vi "GetLowPrioritySensors.vi"() -> ()   [LabVIEW 2023]
doc: "All low priority sensor reads should be placed in this VI."
uses:
  GlobalNoteHandling.vi
  GlobalMiscellaneous.vi
  GlobalDriverStationData.vi
  GlobalDrivebase.vi
  GRNF_CTREMotor.vi
  <vilib>/Rock Robotics/WPI/ThirdParty/Phoenix-LabVIEW/Motor Controller/Get/CTRE_Phoenix_MotorController_GetTemperature.vi
  GRNF_Compressor.vi
  GlobalElevator.vi
  GlobalShooter.vi
  GRNF_GenericMotor.vi
  GRNF_Kraken.vi
  <vilib>/Rock Robotics/WPI/ThirdParty/Phoenix6/getters/GetPRO_SupplyAndTemp_DeviceTemp.vi
  <vilib>/Rock Robotics/WPI/ThirdParty/Phoenix6/getters/GetPRO_RotorPosAndVel_Velocity.vi
panel:
  out "Pressure Change (psi/min)":dbl
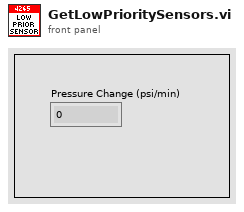
[diagram p1: front panel]
types:
  T1 = typedef "DeviceReference.ctl" = cluster{"CANbus Name":string, "Device Encoding":u32, "Device Name":string}
  T2 = cluster{"Value":dbl, "System Timestamp":dbl, "CANivore Timestamp":dbl, "ECU Timestamp":dbl}
  T3 = typedef "WPI_MotorControlDeviceRef.ctl" = cluster{"DeviceStatus":errorcluster, "Type":T4, "PWM":cluster{"PWM Channel":T5, "DeadBand":T6}, "CAN":cluster{"Device Number":u8, "SetOutput VI Ref":variant, "GetOutput VI Ref":variant, "Enable VI Ref":variant, "Disable VI Ref":variant, "Data":variant}, "Invert":bool, "DIO PWM":cluster{"PWM \"Enable\" Channel":T5, "DIOChannel":T7, "PWM Rate":dbl}}
  T4 = typedef "WPI_MotorControlType.ctl" = enum16{"PWM", "CAN", "DIO PWM"}
  T5 = typedef "FPGA_DIOPWMChannel.ctl" = enum8{"PWM 0", "PWM 1", "PWM 2", "PWM 3", "PWM 4", "PWM 5", "PWM 6", "PWM 7", "PWM 8", "PWM 9", "PWM MXP 0", "PWM MXP 1", "PWM MXP 2", "PWM MXP 3", "PWM MXP 4", "PWM MXP 5", "PWM MXP 6", "PWM MXP 7", "PWM MXP 8", "PWM MXP 9", "Invalid"}
  T6 = typedef "WPI_PWMDeadband.ctl" = cluster{"Name":string, "maxPositivePwm":i32, "minPositivePwm":i32, "centerPwm":i32, "maxNegativePwm":i32, "minNegativePwm":i32, "angularRange":u16}
  T7 = typedef "FPGA_DIOChannel.ctl" = enum8{"DIO 0", "DIO 1", "DIO 2", "DIO 3", "DIO 4", "DIO 5", "DIO 6", "DIO 7", "DIO 8", "DIO 9", "DIO MXP 0", "DIO MXP 1", "DIO MXP 2", "DIO MXP 3", "DIO MXP 4", "DIO MXP 5", "DIO MXP 6", "DIO MXP 7", "DIO MXP 8", "DIO MXP 9", "DIO MXP 10", "DIO MXP 11", "DIO MXP 12", "DIO MXP 13", "DIO MXP 14", "DIO MXP 15", "SPI Port CS1", "SPI Port CS2", "SPI Port CS3", "SPI Port MISO", "SPI Port MOSI", "Invalid"}
  T8 = typedef "WPI_CompressorDevRef.ctl" = cluster{"DevStatus":errorcluster, "Pneumatics Control Module":u8}
  T9 = cluster{"Pressure 0 (psi)":dbl, "Pressure 1 (psi)":dbl}
  T10 = cluster{"Battery Voltage Fault":bool, "Hardware Fault":bool, "CAN Warning Fault":bool, "Temperature Fault":bool}
  T11 = cluster{"HardwareFault":bool, "CompressorFault":bool, "SolenoidFault":bool, "Compressor Open":bool, "Brownout":bool}
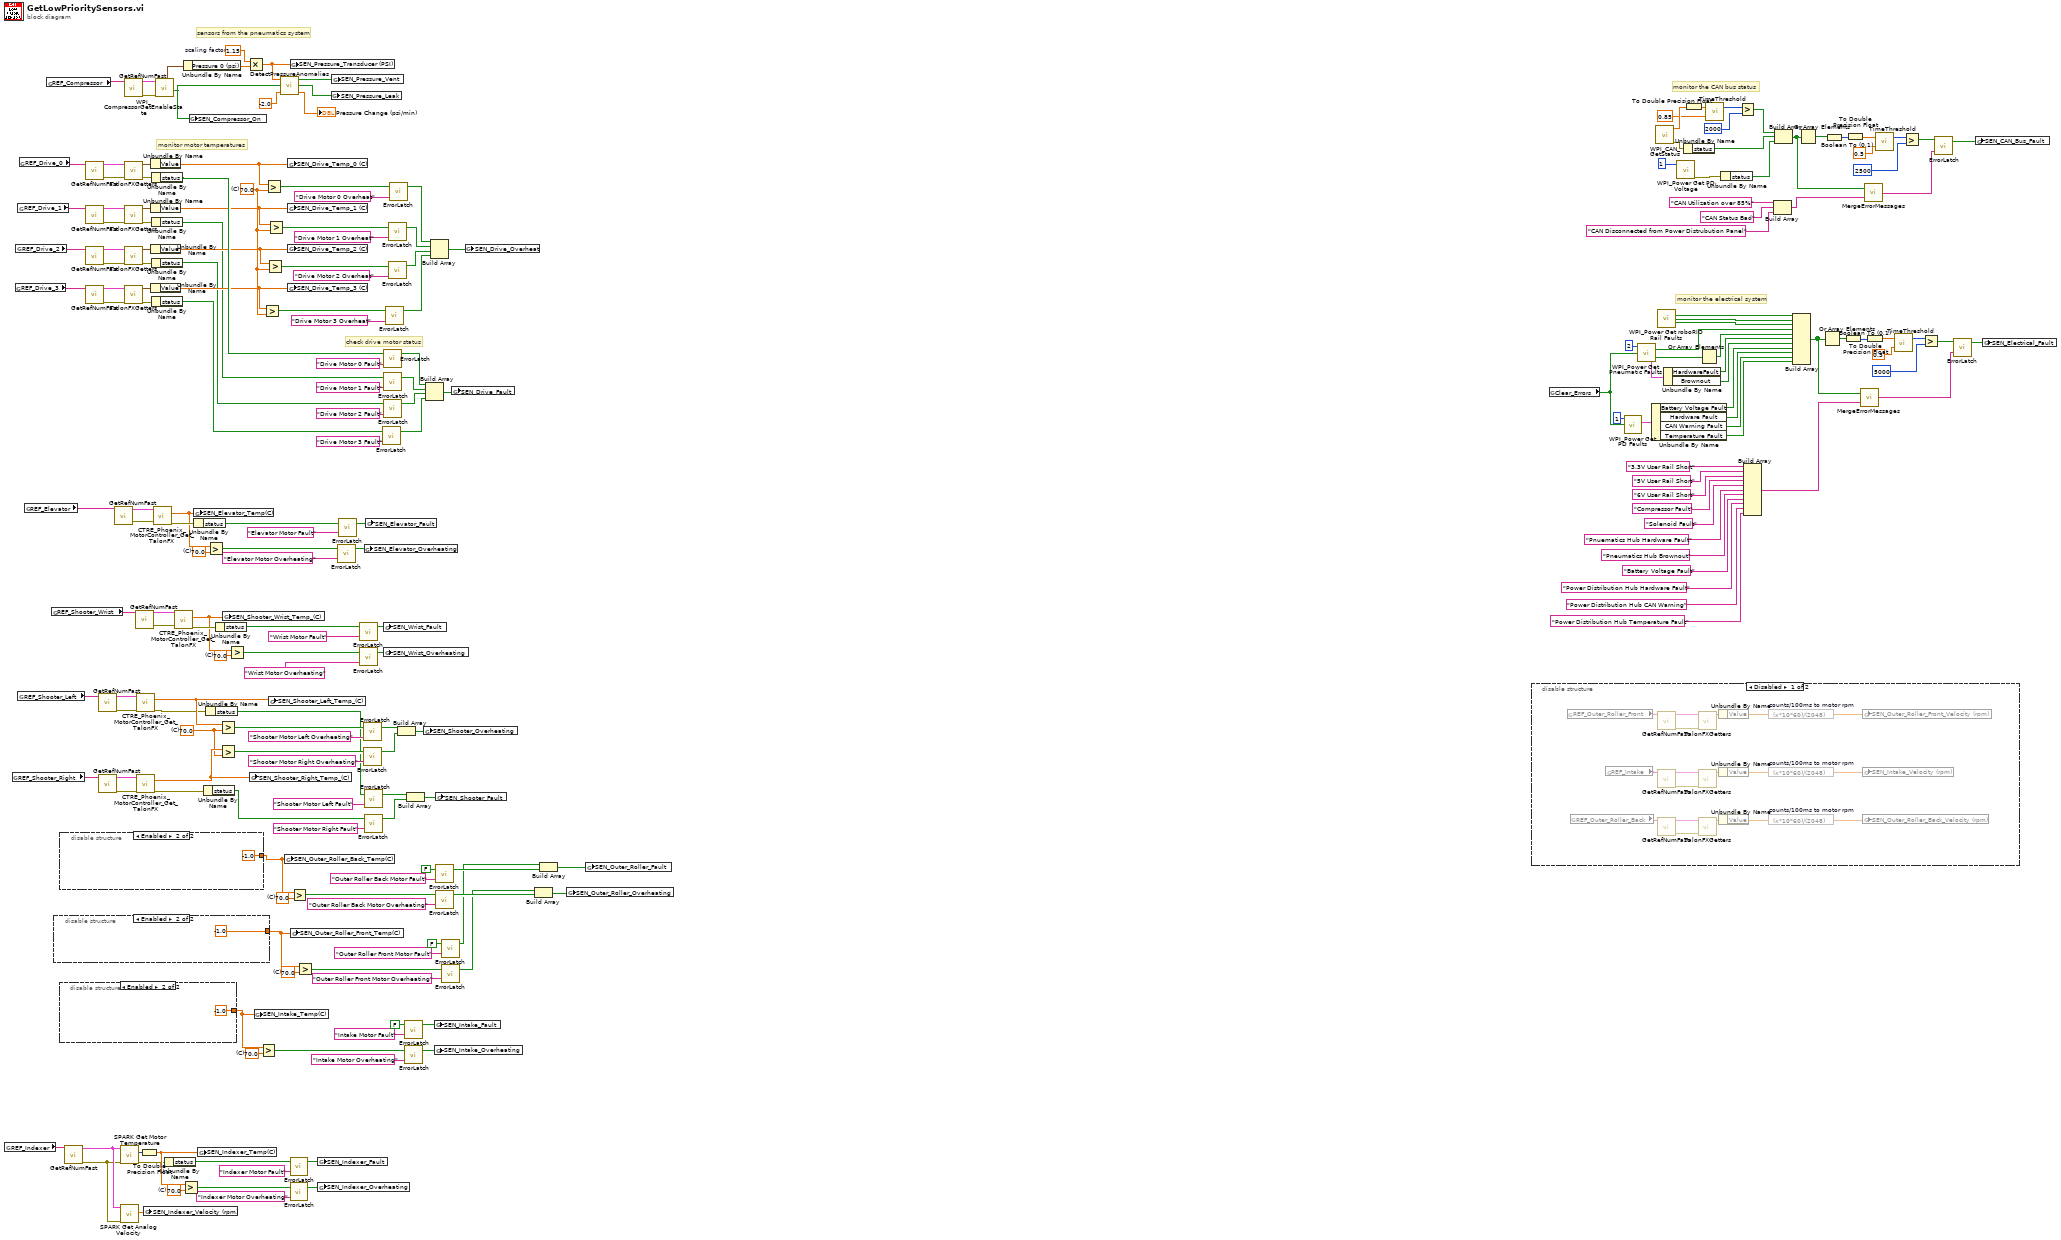
[diagram p0: block diagram]
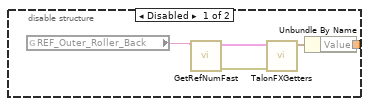
[diagram p3: hidden frame]
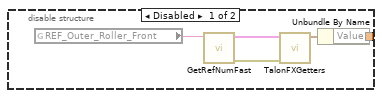
[diagram p4: hidden frame]
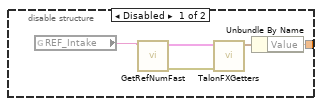
[diagram p5: hidden frame]
diagram:
  w34 = 70.0  # (C)
  w42 = 70.0  # (C)
  w49 = 70.0  # (C)
  w60 = 70.0  # (C)
  w78 = 70.0  # (C)
  w105 = 70.0  # (C)
  w108 = 70.0  # (C)
  w129 = 1.15  # scaling factor
  w216 = 70.0  # (C)
  # "check drive motor status"
  # "monitor the electrical system"
  # "monitor the CAN bus status"
  # "monitor motor temperatures"
  # "sensors from the pneumatics system"
  n1 = global read "GlobalNoteHandling.vi" "REF_Indexer"() -> (w66:string)
  n2 = global read "GlobalShooter.vi" "REF_Shooter_Right"() -> (w69:string)
  n3 = global read "GlobalDrivebase.vi" "REF_Drive_3"() -> (w7:string)
  n4 = global read "GlobalDrivebase.vi" "REF_Drive_2"() -> (w8:string)
  n5 = global read "GlobalDrivebase.vi" "REF_Drive_1"() -> (w9:string)
  n6 = global read "GlobalShooter.vi" "REF_Shooter_Left"() -> (w81:string)
  n7 = global read "GlobalDrivebase.vi" "REF_Drive_0"() -> (w28:string)
  n8 = global read "GlobalElevator.vi" "REF_Elevator"() -> (w114:string)
  n9 = global read "GlobalMiscellaneous.vi" "REF_Compressor"() -> (w175:string)
  n10 = global read "GlobalShooter.vi" "REF_Shooter_Wrist"() -> (w97:string)
  n11 = disable-structure shown="Enabled" {
    disable-tunnel: [w217 -1.0 ("SEN_Intake_Temp(C)")] -> w44
    frame Disabled {
      n12 = global read "GlobalNoteHandling.vi" "REF_Outer_Roller_Front"() -> (w218:string)
      n13 = call-poly "GetRefNumFast.vi"("RefNum Name"=w218) -> ("Error"=w220:errorcluster, "Device Reference"=w219:T1)  [unwired: 5 in]
      n14 = call-poly <vilib>:"TalonFXGetters.vi"("error in"=w220, "DeviceReference"=w219) -> ("Output"=w221:T2)  [unwired: 8 in, 1 out]
      n15 = Unbundle By Name(w221) -> ("Value"=w217:dbl)
    }
    frame Enabled {
    }
  }
  n16 = disable-structure shown="Enabled" {
    disable-tunnel: [w227 -1.0 ("SEN_Intake_Temp(C)")] -> w39
    frame Disabled {
      n17 = global read "GlobalNoteHandling.vi" "REF_Intake"() -> (w226:string)
      n18 = call-poly "GetRefNumFast.vi"("RefNum Name"=w226) -> ("Error"=w224:errorcluster, "Device Reference"=w223:T1)  [unwired: 5 in]
      n19 = call-poly <vilib>:"TalonFXGetters.vi"("error in"=w224, "DeviceReference"=w223) -> ("Output"=w225:T2)  [unwired: 8 in, 1 out]
      n20 = Unbundle By Name(w225) -> ("Value"=w227:dbl)
    }
    frame Enabled {
    }
  }
  n21 = disable-structure shown="Enabled" {
    disable-tunnel: [w229 -1.0 ("SEN_Outer_Roller_Back_Temp(C)")] -> w51
    frame Disabled {
      n22 = global read "GlobalNoteHandling.vi" "REF_Outer_Roller_Back"() -> (w230:string)
      n23 = call-poly "GetRefNumFast.vi"("RefNum Name"=w230) -> ("Error"=w232:errorcluster, "Device Reference"=w233:T1)  [unwired: 5 in]
      n24 = call-poly <vilib>:"TalonFXGetters.vi"("error in"=w232, "DeviceReference"=w233) -> ("Output"=w231:T2)  [unwired: 8 in, 1 out]
      n25 = Unbundle By Name(w231) -> ("Value"=w229:dbl)
    }
    frame Enabled {
    }
  }
  n26 = call-poly "GetRefNumFast.vi"("RefNum Name"=w66) -> ("Error"=w54:errorcluster, "Device Reference"=w55:T3)  [unwired: 5 in]
  n27 = call-poly "GetRefNumFast.vi"("RefNum Name"=w28) -> ("Error"=w26:errorcluster, "Device Reference"=w27:T1)  [unwired: 5 in]
  n28 = call-poly "GetRefNumFast.vi"("RefNum Name"=w9) -> ("Error"=w19:errorcluster, "Device Reference"=w18:T1)  [unwired: 5 in]
  n29 = call-poly "GetRefNumFast.vi"("RefNum Name"=w8) -> ("Error"=w16:errorcluster, "Device Reference"=w17:T1)  [unwired: 5 in]
  n30 = call-poly "GetRefNumFast.vi"("RefNum Name"=w7) -> ("Error"=w11:errorcluster, "Device Reference"=w10:T1)  [unwired: 5 in]
  n31 = call-poly "GetRefNumFast.vi"("RefNum Name"=w81) -> ("Error"=w75:errorcluster, "Device Reference"=w74:T3)  [unwired: 5 in]
  n32 = call-poly "GetRefNumFast.vi"("RefNum Name"=w69) -> ("Error"=w70:errorcluster, "Device Reference"=w71:T3)  [unwired: 5 in]
  n33 = call-poly "GetRefNumFast.vi"("RefNum Name"=w114) -> ("Error"=w116:errorcluster, "Device Reference"=w115:T3)  [unwired: 5 in]
  n34 = call <vilib>:"SPARK Get Analog Velocity.vi"("error in (no error)"=w54, "MotorControlDevRef in"=w55) -> ("Analog Velocity"=w53:dbl)  [unwired: 6 in, 3 out]
  n35 = call <vilib>:"SPARK Get Motor Temperature.vi"("error in (no error)"=w54, "MotorControlDevRef in"=w55) -> ("error out"=w57:errorcluster, "Motor Temperature"=w59:u8)  [unwired: 6 in, 2 out]
  n36 = call-poly "GetRefNumFast.vi"("RefNum Name"=w175) -> ("Error"=w199:errorcluster, "Device Reference"=w200:T8)  [unwired: 5 in]
  n37 = call-poly <vilib>:"TalonFXGetters.vi"("error in"=w26, "DeviceReference"=w27) -> ("error out"=w25:errorcluster, "Output"=w23:T2)  [unwired: 8 in]
  n38 = call-poly <vilib>:"TalonFXGetters.vi"("error in"=w19, "DeviceReference"=w18) -> ("error out"=w20:errorcluster, "Output"=w21:T2)  [unwired: 8 in]
  n39 = call-poly <vilib>:"TalonFXGetters.vi"("error in"=w16, "DeviceReference"=w17) -> ("error out"=w15:errorcluster, "Output"=w14:T2)  [unwired: 8 in]
  n40 = call-poly <vilib>:"TalonFXGetters.vi"("error in"=w11, "DeviceReference"=w10) -> ("error out"=w12:errorcluster, "Output"=w13:T2)  [unwired: 8 in]
  n41 = call-poly "GetRefNumFast.vi"("RefNum Name"=w97) -> ("Error"=w99:errorcluster, "Device Reference"=w100:T3)  [unwired: 5 in]
  n42 = call-poly <vilib>:"CTRE_Phoenix_MotorController_Get_TalonFX.vi"("PhoenixMotorControlDevRef"=w74, "error in"=w75) -> ("Temperature (C)"=w80:dbl, "error out"=w73:errorcluster)  [unwired: 11 in, 1 out]
  n43 = call-poly <vilib>:"CTRE_Phoenix_MotorController_Get_TalonFX.vi"("PhoenixMotorControlDevRef"=w71, "error in"=w70) -> ("Temperature (C)"=w79:dbl, "error out"=w68:errorcluster)  [unwired: 11 in, 1 out]
  n44 = To Double Precision Float(number=w59) -> (double precision float=w58:dbl)
  n45 = global write "GlobalNoteHandling.vi" "SEN_Indexer_Velocity (rpm)"(w53) -> ()
  n46 = Unbundle By Name(w23) -> ("Value"=w22:dbl)
  n47 = Unbundle By Name(w21) -> ("Value"=w5:dbl)
  n48 = Unbundle By Name(w14) -> ("Value"=w4:dbl)
  n49 = Unbundle By Name(w13) -> ("Value"=w6:dbl)
  n50 = Unbundle By Name(w25) -> ("status"=w24:bool)
  n51 = Unbundle By Name(w20) -> ("status"=w2:bool)
  n52 = Unbundle By Name(w15) -> ("status"=w3:bool)
  n53 = Unbundle By Name(w12) -> ("status"=w1:bool)
  n54 = call-poly <vilib>:"CTRE_Phoenix_MotorController_Get_TalonFX.vi"("PhoenixMotorControlDevRef"=w115, "error in"=w116) -> ("Temperature (C)"=w109:dbl, "error out"=w117:errorcluster)  [unwired: 11 in, 1 out]
  n55 = call <vilib>:"WPI_CompressorGetEnableState.vi"("error in (no error)"=w199, "CompressorDevRef"=w200) -> ("Compressor Running"=w172:bool, "Pressure Sensors"=w181:T9)  [unwired: 3 in, 5 out]
  n56 = Unbundle By Name(w57) -> ("status"=w56:bool)
  n57 = call-poly <vilib>:"CTRE_Phoenix_MotorController_Get_TalonFX.vi"("PhoenixMotorControlDevRef"=w100, "error in"=w99) -> ("Temperature (C)"=w96:dbl, "error out"=w98:errorcluster)  [unwired: 11 in, 1 out]
  n58 = Greater?(x=w58, y=w60) -> (0:w61:bool)
  n59 = Unbundle By Name(w181) -> ("Pressure 0 (psi)"=w131:dbl)
  n60 = global write "GlobalMiscellaneous.vi" "SEN_Compressor_On"(w172) -> ()
  n61 = global write "GlobalElevator.vi" "SEN_Elevator_Temp(C)"(w109) -> ()
  n62 = Unbundle By Name(w117) -> ("status"=w112:bool)
  n63 = global write "GlobalNoteHandling.vi" "SEN_Indexer_Temp(C)"(w58) -> ()
  n64 = Unbundle By Name(w68) -> ("status"=w67:bool)
  n65 = Unbundle By Name(w73) -> ("status"=w72:bool)
  n66 = Greater?(x=w109, y=w108) -> (0:w110:bool)
  n67 = Unbundle By Name(w98) -> ("status"=w102:bool)
  n68 = Greater?(x=w80, y=w78) -> (0:w89:bool)
  n69 = Greater?(x=w79, y=w78) -> (0:w91:bool)
  n70 = global write "GlobalShooter.vi" "SEN_Shooter_Wrist_Temp_(C)"(w96) -> ()
  n71 = Greater?(x=w96, y=w105) -> (0:w104:bool)
  n72 = Multiply(x=w129, y=w131) -> (x*y=w130:dbl)
  n73 = global write "GlobalShooter.vi" "SEN_Shooter_Right_Temp_(C)"(w79) -> ()
  n74 = global write "GlobalNoteHandling.vi" "SEN_Intake_Temp(C)"(w39) -> ()
  n75 = Greater?(x=w39, y=w34) -> (0:w36:bool)
  n76 = Greater?(x=w6, y=w216) -> (0:w133:bool)
  n77 = Greater?(x=w22, y=w216) -> (0:w143:bool)
  n78 = Greater?(x=w4, y=w216) -> (0:w136:bool)
  n79 = Greater?(x=w5, y=w216) -> (0:w139:bool)
  n80 = global write "GlobalShooter.vi" "SEN_Shooter_Left_Temp_(C)"(w80) -> ()
  n81 = call "DetectPressureAnomalies.vi"("Pressure Loss Threshold (psi/min)"=-2.0, "Compressor Running"=w172, "Pressure (psi)"=w130) -> ("Pressure Change (psi/min)"=→"Pressure Change (psi/min)":dbl, "Pressure Leak"=w173:bool, "Pressure Vent"=w174:bool)
  n82 = global write "GlobalNoteHandling.vi" "SEN_Outer_Roller_Back_Temp(C)"(w51) -> ()
  n83 = global write "GlobalDrivebase.vi" "SEN_Drive_Temp_0 (C)"(w22) -> ()
  n84 = global write "GlobalDrivebase.vi" "SEN_Drive_Temp_1 (C)"(w5) -> ()
  n85 = global write "GlobalDrivebase.vi" "SEN_Drive_Temp_2 (C)"(w4) -> ()
  n86 = global write "GlobalDrivebase.vi" "SEN_Drive_Temp_3 (C)"(w6) -> ()
  n87 = global write "GlobalMiscellaneous.vi" "SEN_Pressure_Transducer (PSI)"(w130) -> ()
  n88 = call "ErrorLatch.vi"("Error Message"="Indexer Motor Fault", "Trigger"=w56) -> ("Latched"=w65:bool)  [unwired: 1 in]
  n89 = call "ErrorLatch.vi"("Error Message"="Indexer Motor Overheating", "Trigger"=w61) -> ("Latched"=w64:bool)  [unwired: 1 in]
  n90 = Greater?(x=w51, y=w49) -> (0:w52:bool)
  n91 = global write "GlobalNoteHandling.vi" "SEN_Outer_Roller_Front_Temp(C)"(w44) -> ()
  n92 = Greater?(x=w44, y=w42) -> (0:w45:bool)
  n93 = global write "GlobalNoteHandling.vi" "SEN_Indexer_Fault"(w65) -> ()
  n94 = global write "GlobalNoteHandling.vi" "SEN_Indexer_Overheating"(w64) -> ()
  n95 = global write "GlobalMiscellaneous.vi" "SEN_Pressure_Leak"(w173) -> ()
  n96 = global write "GlobalMiscellaneous.vi" "SEN_Pressure_Vent"(w174) -> ()
  n97 = call "ErrorLatch.vi"("Error Message"="Elevator Motor Overheating", "Trigger"=w110) -> ("Latched"=w106:bool)  [unwired: 1 in]
  n98 = call "ErrorLatch.vi"("Error Message"="Elevator Motor Fault", "Trigger"=w112) -> ("Latched"=w107:bool)  [unwired: 1 in]
  n99 = call "ErrorLatch.vi"("Error Message"="Wrist Motor Overheating", "Trigger"=w104) -> ("Latched"=w95:bool)  [unwired: 1 in]
  n100 = call "ErrorLatch.vi"("Error Message"="Wrist Motor Fault", "Trigger"=w102) -> ("Latched"=w94:bool)  [unwired: 1 in]
  n101 = call "ErrorLatch.vi"("Error Message"="Shooter Motor Left Overheating", "Trigger"=w89) -> ("Latched"=w90:bool)  [unwired: 1 in]
  n102 = call "ErrorLatch.vi"("Error Message"="Shooter Motor Right Overheating", "Trigger"=w91) -> ("Latched"=w93:bool)  [unwired: 1 in]
  n103 = global write "GlobalElevator.vi" "SEN_Elevator_Overheating"(w106) -> ()
  n104 = call "ErrorLatch.vi"("Error Message"="Shooter Motor Left Fault", "Trigger"=w72) -> ("Latched"=w85:bool)  [unwired: 1 in]
  n105 = call "ErrorLatch.vi"("Error Message"="Shooter Motor Right Fault", "Trigger"=w67) -> ("Latched"=w87:bool)  [unwired: 1 in]
  n106 = global write "GlobalElevator.vi" "SEN_Elevator_Fault"(w107) -> ()
  n107 = call "ErrorLatch.vi"("Error Message"="Drive Motor 3 Fault", "Trigger"=w1) -> ("Latched"=w121:bool)  [unwired: 1 in]
  n108 = global write "GlobalShooter.vi" "SEN_Wrist_Fault"(w94) -> ()
  n109 = global write "GlobalShooter.vi" "SEN_Wrist_Overheating"(w95) -> ()
  n110 = call "ErrorLatch.vi"("Error Message"="Drive Motor 0 Fault", "Trigger"=w24) -> ("Latched"=w125:bool)  [unwired: 1 in]
  n111 = call "ErrorLatch.vi"("Error Message"="Drive Motor 1 Fault", "Trigger"=w2) -> ("Latched"=w124:bool)  [unwired: 1 in]
  n112 = call "ErrorLatch.vi"("Error Message"="Drive Motor 2 Fault", "Trigger"=w3) -> ("Latched"=w123:bool)  [unwired: 1 in]
  n113 = call "ErrorLatch.vi"("Error Message"="Drive Motor 3 Overheat", "Trigger"=w133) -> ("Latched"=w132:bool)  [unwired: 1 in]
  n114 = call "ErrorLatch.vi"("Error Message"="Drive Motor 2 Overheat", "Trigger"=w136) -> ("Latched"=w135:bool)  [unwired: 1 in]
  n115 = call "ErrorLatch.vi"("Error Message"="Drive Motor 1 Overheat", "Trigger"=w139) -> ("Latched"=w138:bool)  [unwired: 1 in]
  n116 = call "ErrorLatch.vi"("Error Message"="Drive Motor 0 Overheat", "Trigger"=w143) -> ("Latched"=w142:bool)  [unwired: 1 in]
  n117 = Build Array(w90, w93) -> (w83:bool[])
  n118 = call "ErrorLatch.vi"("Error Message"="Intake Motor Fault", "Trigger"=FALSE) -> ("Latched"=w38:bool)  [unwired: 1 in]
  n119 = call "ErrorLatch.vi"("Error Message"="Intake Motor Overheating", "Trigger"=w36) -> ("Latched"=w37:bool)  [unwired: 1 in]
  n120 = Build Array(w85, w87) -> (w82:bool[])
  n121 = global write "GlobalShooter.vi" "SEN_Shooter_Overheating"(w83) -> ()
  n122 = Build Array(w125, w124, w123, w121) -> (w120:bool[])
  n123 = Build Array(w142, w138, w135, w132) -> (w144:bool[])
  n124 = global write "GlobalNoteHandling.vi" "SEN_Intake_Fault"(w38) -> ()
  n125 = global write "GlobalNoteHandling.vi" "SEN_Intake_Overheating"(w37) -> ()
  n126 = global write "GlobalShooter.vi" "SEN_Shooter_Fault"(w82) -> ()
  n127 = call "ErrorLatch.vi"("Error Message"="Outer Roller Back Motor Fault", "Trigger"=FALSE) -> ("Latched"=w46:bool)  [unwired: 1 in]
  n128 = call "ErrorLatch.vi"("Error Message"="Outer Roller Back Motor Overheating", "Trigger"=w52) -> ("Latched"=w47:bool)  [unwired: 1 in]
  n129 = call "ErrorLatch.vi"("Error Message"="Outer Roller Front Motor Fault", "Trigger"=FALSE) -> ("Latched"=w40:bool)  [unwired: 1 in]
  n130 = call "ErrorLatch.vi"("Error Message"="Outer Roller Front Motor Overheating", "Trigger"=w45) -> ("Latched"=w32:bool)  [unwired: 1 in]
  n131 = global write "GlobalDrivebase.vi" "SEN_Drive_Fault"(w120) -> ()
  n132 = global write "GlobalDrivebase.vi" "SEN_Drive_Overheat"(w144) -> ()
  n133 = Build Array(w32, w47) -> (w76:bool[])
  n134 = Build Array(w40, w46) -> (w77:bool[])
  n135 = global write "GlobalNoteHandling.vi" "SEN_Outer_Roller_Overheating"(w76) -> ()
  n136 = global write "GlobalNoteHandling.vi" "SEN_Outer_Roller_Fault"(w77) -> ()
  n137 = disable-structure shown="Disabled" {
    frame Disabled {
      n138 = global read "GlobalNoteHandling.vi" "REF_Outer_Roller_Front"() -> (w246:string)
      n139 = global read "GlobalNoteHandling.vi" "REF_Outer_Roller_Back"() -> (w238:string)
      n140 = global read "GlobalNoteHandling.vi" "REF_Intake"() -> (w237:string)
      n141 = call-poly "GetRefNumFast.vi"("RefNum Name"=w246) -> ("Error"=w248:errorcluster, "Device Reference"=w247:T1)  [unwired: 5 in]
      n142 = call-poly "GetRefNumFast.vi"("RefNum Name"=w237) -> ("Error"=w243:errorcluster, "Device Reference"=w244:T1)  [unwired: 5 in]
      n143 = call-poly "GetRefNumFast.vi"("RefNum Name"=w238) -> ("Error"=w240:errorcluster, "Device Reference"=w239:T1)  [unwired: 5 in]
      n144 = call-poly <vilib>:"TalonFXGetters.vi"("error in"=w248, "DeviceReference"=w247) -> ("Output"=w249:T2)  [unwired: 8 in, 1 out]
      n145 = call-poly <vilib>:"TalonFXGetters.vi"("error in"=w243, "DeviceReference"=w244) -> ("Output"=w242:T2)  [unwired: 8 in, 1 out]
      n146 = call-poly <vilib>:"TalonFXGetters.vi"("error in"=w240, "DeviceReference"=w239) -> ("Output"=w241:T2)  [unwired: 8 in, 1 out]
      n147 = Unbundle By Name(w249) -> ("Value"=w245:dbl)
      n148 = Unbundle By Name(w242) -> ("Value"=w235:dbl)
      n149 = Unbundle By Name(w241) -> ("Value"=w236:dbl)
      n150 = expression code="(x*10*60)/(2048)" "counts/100ms to motor rpm"(w245) -> (w252:dbl)
      n151 = expression code="(x*10*60)/(2048)" "counts/100ms to motor rpm"(w235) -> (w251:dbl)
      n152 = expression code="(x*10*60)/(2048)" "counts/100ms to motor rpm"(w236) -> (w250:dbl)
      n153 = global write "GlobalNoteHandling.vi" "SEN_Outer_Roller_Front_Velocity (rpm)"(w252) -> ()
      n154 = global write "GlobalNoteHandling.vi" "SEN_Intake_Velocity (rpm)"(w251) -> ()
      n155 = global write "GlobalNoteHandling.vi" "SEN_Outer_Roller_Back_Velocity (rpm)"(w250) -> ()
    }
    frame Enabled {
    }
  }
  n156 = global read "GlobalDriverStationData.vi" "Clear_Errors"() -> (w182:bool)
  n157 = call <vilib>:"WPI_Power Get PD Faults.vi"("Power Distribution (def)"=u8 1, "Clear Sticky Faults"=w182) -> ("Faults"=w192:T10)  [unwired: 10 in, 3 out]
  n158 = call <vilib>:"WPI_Power Get Pneumatic Faults.vi"("Pneumatics device (def)"=u8 2, "Clear Sticky Faults"=w182) -> ("Compressor Fault"=w197:bool, "All Solenoid Faults"=w196:bool[], "Faults"=w188:T11)  [unwired: 8 in, 3 out]
  n159 = Unbundle By Name(w192) -> ("Battery Voltage Fault"=w145:bool, "Hardware Fault"=w185:bool, "CAN Warning Fault"=w184:bool, "Temperature Fault"=w183:bool)
  n160 = call <vilib>:"WPI_CAN_GetStatus.vi"() -> ("error out"=w214:errorcluster, "Percent Bus Utilization"=w211:sgl)  [unwired: 6 in, 4 out]
  n161 = call <vilib>:"WPI_Power Get roboRIO Rail Faults.vi"() -> ("3.3V User Rail Short"=w195:bool, "5 V User Rail Short"=w194:bool, "6 V User Rail Short"=w193:bool)  [unwired: 10 in, 3 out]
  n162 = Unbundle By Name(w188) -> ("HardwareFault"=w187:bool, "Brownout"=w186:bool)
  n163 = call <vilib>:"WPI_Power Get PD Voltage.vi"("Power Distribution Panel (def)"=u8 1 ("Power Distribution Panel (0)")) -> ("error out"=w190:errorcluster)  [unwired: 13 in, 1 out]
  n164 = Unbundle By Name(w214) -> ("status"=w213:bool)
  n165 = To Double Precision Float(number=w211) -> (double precision float=w209:dbl)
  n166 = Or Array Elements(Boolean array=w196) -> (logical OR=w215:bool)
  n167 = call "TimeThreshold.vi"("Threshold"=0.85, "Current Value"=w209) -> ("Time Above Threshold (ms)"=w208:u32)  [unwired: 1 out]
  n168 = Unbundle By Name(w190) -> ("status"=w212:bool)
  n169 = Greater?(x=w208, y=u32 2000) -> (0:w118:bool)
  n170 = Build Array("3.3V User Rail Short", "5V User Rail Short" ("element"), "6V User Rail Short" ("element"), "Compressor Fault" ("element"), "Solenoid Fault" ("element"), "Pnuematics Hub Hardware Fault" ("element"), "Pneumatics Hub Brownout" ("element"), "Battery Voltage Fault" ("element"), "Power Distribution Hub Hardware Fault" ("element"), "Power Distribution Hub CAN Warning" ("element"), "Power Distribution Hub Temperature Fault" ("element")) -> (w150:string[])
  n171 = Build Array("CAN Utilization over 85%", "CAN Status Bad" ("element"), "CAN Disconnected from Power Distrubution Panel" ("element")) -> (w146:string[])
  n172 = Build Array(w118, w213, w212) -> (w147:bool[])
  n173 = Build Array(w195, w194, w193, w197, w215, w187, w186, w145, w185, w184, w183) -> (w149:bool[])
  n174 = Or Array Elements(Boolean array=w147) -> (logical OR=w151:bool)
  n175 = Or Array Elements(Boolean array=w149) -> (logical OR=w169:bool)
  n176 = Boolean To (0,1)(Boolean=w151) -> (0, 1=w180:i16)
  n177 = Boolean To (0,1)(Boolean=w169) -> (0, 1=w207:i16)
  n178 = To Double Precision Float(number=w180) -> (double precision float=w179:dbl)
  n179 = call "MergeErrorMessages.vi"("Error Descriptions"=w150, "Active Errors"=w149) -> ("Merged Error Message"=w157:string)
  n180 = call "MergeErrorMessages.vi"("Error Descriptions"=w146, "Active Errors"=w147) -> ("Merged Error Message"=w148:string)
  n181 = To Double Precision Float(number=w207) -> (double precision float=w206:dbl)
  n182 = call "TimeThreshold.vi"("Threshold"=0.5, "Current Value"=w179) -> ("Time Above Threshold (ms)"=w177:u32)  [unwired: 1 out]
  n183 = call "TimeThreshold.vi"("Threshold"=0.5, "Current Value"=w206) -> ("Time Above Threshold (ms)"=w204:u32)  [unwired: 1 out]
  n184 = Greater?(x=w177, y=u32 2500) -> (0:w153:bool)
  n185 = Greater?(x=w204, y=u32 5000) -> (0:w171:bool)
  n186 = call "ErrorLatch.vi"("Error Message"=w148, "Trigger"=w153) -> ("Latched"=w152:bool)  [unwired: 1 in]
  n187 = call "ErrorLatch.vi"("Error Message"=w157, "Trigger"=w171) -> ("Latched"=w170:bool)  [unwired: 1 in]
  n188 = global write "GlobalMiscellaneous.vi" "SEN_CAN_Bus_Fault"(w152) -> ()
  n189 = global write "GlobalMiscellaneous.vi" "SEN_Electrical_Fault"(w170) -> ()
